vi "(Global) Current handle and LaserPower_YCC.vi"() -> ()   [LabVIEW 2014]
panel:
  out "Current PD (mV)":dbl
  out "Current handle":i32
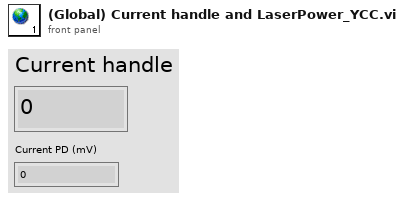
[diagram p1: front panel]
diagram:
